vi "Read time to plot.vi"(8 "error in (no error)":errorcluster, 11 "NIringPlotHandle in":refnum<class "NIringPlotHandle.lvclass">) -> (0 "error out":errorcluster, 2 "time to plot":refnum<user-event>, 3 "NIringPlotHandle out":refnum<class "NIringPlotHandle.lvclass">)   [LabVIEW 2021, in "NIringPlotHandle.lvclass"]
uses:
  NIringPlotHandle.lvclass
  NIringPlotHandle.lvclass/NIringPlotHandle.ctl
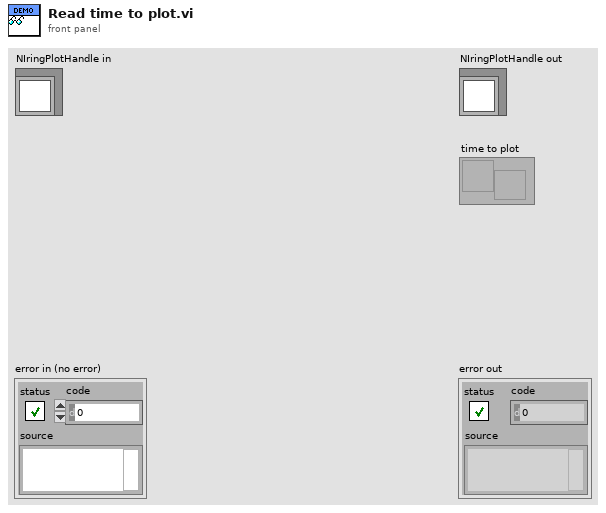
[diagram p1: front panel]
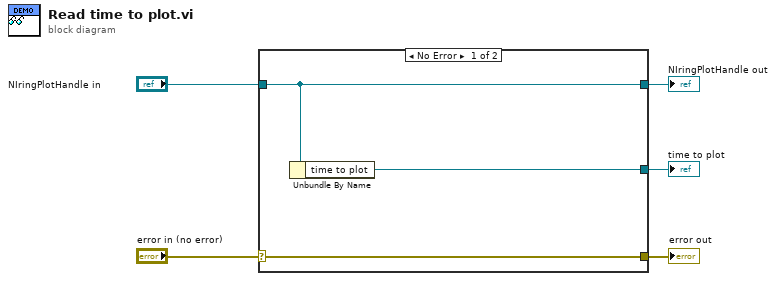
[diagram p0: block diagram]
diagram:
  n1 = case shown="No Error" "error in (no error)" {
    selector: "error in (no error)" -> [w8 w9]
    tunnel: [w8 w9] -> w4
    tunnel: [w7 w10] -> w2
    tunnel: "NIringPlotHandle in" -> [w7 w10]
    tunnel: [w6 _] -> w1
    frame No Error {
      n2 = Unbundle By Name(w7) -> ("time to plot"=w6:refnum<user-event>)
    }
    frame Error {
    }
  }
  "error out" <- w4
  "NIringPlotHandle out" <- w2
  "time to plot" <- w1
